vi "Items Count.vi"(8 "错误输入":errorcluster, 11 "Listbox Ref":refnum<vi>) -> (0 "错误输出":errorcluster, 2 "Count":i32, 3 "Dup Listbox Ref":refnum<vi>)   [LabVIEW 2011, in "Listbox Tool.lvlib"]
uses:
  Listbox Tool.lvlib
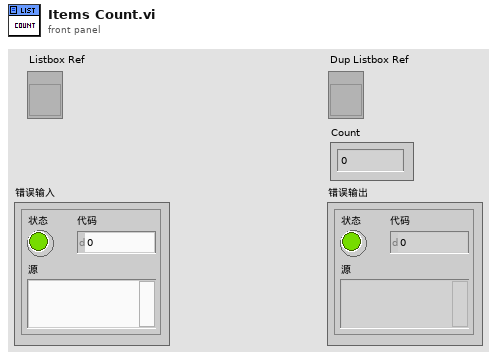
[diagram p1: front panel]
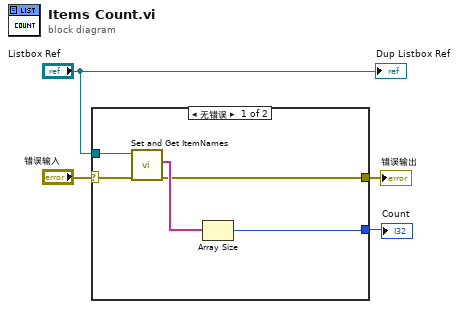
[diagram p0: block diagram]
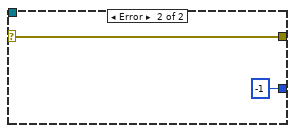
[diagram p2: hidden frame]
diagram:
  n1 = case shown="无错误" "错误输入" {
    selector: "错误输入" -> [w9 w11]
    tunnel: "Listbox Ref" -> [w8 _]
    tunnel: [w6 w11] -> w2
    tunnel: [w5 -1] -> w1
    frame No Error {
      n2 = call "Set and Get ItemNames.vi"("错误输入"=w9, "Listbox Ref"=w8) -> ("错误输出"=w6:errorcluster, "ItemNames Out"=w7:string[])  [unwired: 7 in, 1 out]
      n3 = Array Size(array=w7) -> (size(s)=w5:i32)
    }
    frame Error {
    }
  }
  "错误输出" <- w2
  "Count" <- w1
  "Dup Listbox Ref" <- "Listbox Ref"
